vi "Maximum Amplitude Read.vi"(4 "error in (no error)":errorcluster, 6 "Container State":T2, 7 "Display State In":T1) -> (0 "error out":errorcluster, 2 "Value":dbl, 3 "Display State Out":T1)   [LabVIEW 2017, in "Test Signal Configuration.xctl"]
uses:
  <vilib>/addons/_XControls/Function Generator Configuration/Test Signal Configuration.xctl
  <vilib>/_xctls/Container State.ctl
  <vilib>/addons/_XControls/Function Generator Configuration/Controls/State.ctl
  <vilib>/_xctls/XControlSupport.lvlib
panel:
  # "Replace the Value Indicator below with an Indicator of desired type.\nDo not remove this Indicator or the others from the connector pane. \nDo not change the connector pane pattern.\nThe Value Indicator should always be the second terminal from top on the output side in the connector pane."
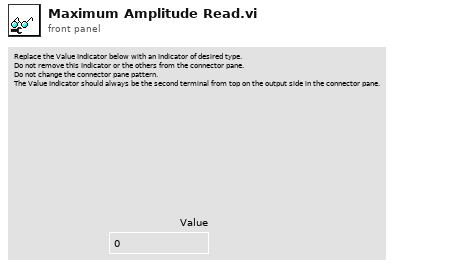
[diagram p1: front panel]
types:
  T1 = typedef "Test Signal Configuration.xctl/State.ctl" = cluster{"Attributes":variant}
  T2 = typedef "XControlSupport.lvlib/Container State.ctl" = cluster{"Indicator?":bool, "Run Mode?":bool, " Refnum":refnum<vi>}
  T3 = typedef "Test Signal Configuration.xctl/signal type.ctl" = enum32{"None", "Tone", "Multitone", "Discrete Sweep", "Continuous Sweep", "Noise"}
  T4 = cluster{"Signal":cluster{"Sample Rate":cluster{"name":string, "default":dbl}, "Signal Type":cluster{"name":string, "signal type":T3}, "Amplitude":cluster{"name":string, "default":dbl}, "Offset":cluster{"name":string, "default":dbl}}, "Function":cluster{"Info":cluster{"name":string, "default":variant}, "Type":cluster{"name":string, "default":u16}, "Frequency":cluster{"name":string, "default":dbl}, "Phase":cluster{"name":string, "default":dbl}}, "Continuous Sweep":cluster{"Info":cluster{"name":string, "default":variant}, "Start":cluster{"name":string, "default":dbl}, "Stop":cluster{"name":string, "default":dbl}, "Duration":cluster{"name":string, "default":dbl}, "Profile":cluster{"name":string, "default":enum16{"Linear", "Logarithmic"}}}, "Discrete Sweep":cluster{"Info":cluster{"name":string, "default":variant}, "Start":cluster{"name":string, "default":dbl}, "Stop":cluster{"name":string, "default":dbl}, "Cycles":cluster{"name":string, "default":dbl}, "Time":cluster{"name":string, "default":dbl}, "Spacing":cluster{"name":string, "default":enum16{"Linear", "Logarithmic"}}, "Steps":cluster{"name":string, "default":i32}}, "Multitone":cluster{"Info":cluster{"name":string, "multitone info":cluster{"frequency":dbl, "amplitude":dbl, "phase":dbl}[]}}, "Noise":cluster{"Info":cluster{"name":string, "default":variant}, "Type":cluster{"name":string, "default":u16}, "Amplitude PDF":cluster{"name":string, "default":enum16{"Gaussian", "Rectangular", "Triangular"}}, "Level":cluster{"name":string, "default":dbl}, "Seed":cluster{"name":string, "default":i32}}, "Configuration":cluster{"Min Frequency":cluster{"name":string, "default":dbl}, "Max Frequency":cluster{"name":string, "default":dbl}, "Max Amplitude":cluster{"name":string, "default":dbl}}}
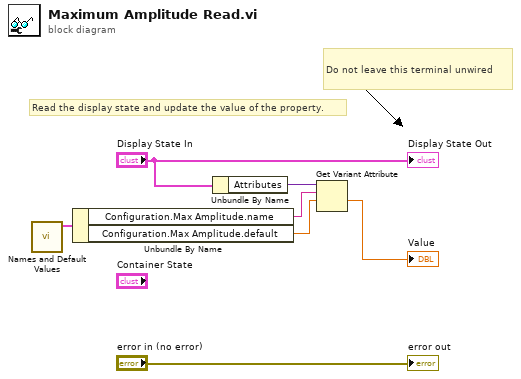
[diagram p0: block diagram]
diagram:
  # "Do not leave this terminal unwired"
  # "Read the display state and update the value of the property."
  n1 = call <vilib>:"Names and Default Values.vi"() -> ("Names and Default Values"=w6:T4)  [unwired: 11 in]
  n2 = Unbundle By Name(w6) -> ("Configuration.Max Amplitude.name"=w3:string, "Configuration.Max Amplitude.default"=w2:dbl)
  n3 = Unbundle By Name("Display State In") -> ("Attributes"=w4:variant)
  n4 = Get Variant Attribute(Variant=w4, name=w3, default value (empty Variant)=w2) -> (value=→"Value":dbl)  [unwired: 1 in, 3 out]
  "error out" <- "error in (no error)"
  "Display State Out" <- "Display State In"
